vi "setMode.vi"(8 "error in (no error)":errorcluster, 10 "mode":T1, 11 "DmmKeysight in":refnum<class "DmmKeysight.lvclass">) -> (0 "error out":errorcluster, 3 "DmmKeysight out":refnum<class "DmmKeysight.lvclass">)   [LabVIEW 2023, in "DmmKeysight.lvclass"]
doc: "<b>Author:</b> Wolfgang\n<b>Description:</b>Define measurement mode: Voltage, Current, Resistance"
uses:
  DmmKeysight.lvclass
  Data/DmmModes.ctl
  Driver/TypeDef/mode.ctl
  DmmKeysight.lvclass/DmmKeysight.ctl
  Multimeter.lvclass
  Driver/Keysight-34450A.lvlib
  sweDmm.lvlib
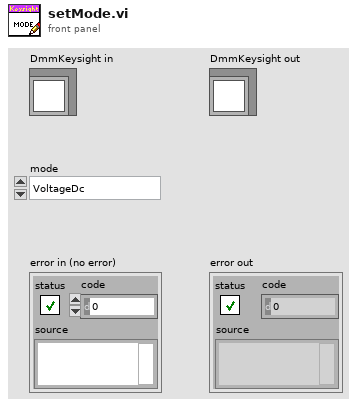
[diagram p1: front panel]
types:
  T1 = typedef "sweDmm.lvlib/DmmModes.ctl" = enum16{"VoltageDc", "VoltageAc", "CurrentDc", "CurrentAc", "Resistance2W"}
  T2 = typedef "Keysight-34450A.lvlib/mode.ctl" = enum16{"DC_Voltage", "AC_Voltage", "DC_Current", "AC_Current", "Resistance"}
  T3 = typedef "Keysight-34450A.lvlib/configuration.ctl" = cluster{"mode":T2, "Range":dbl, "Resolution":dbl}
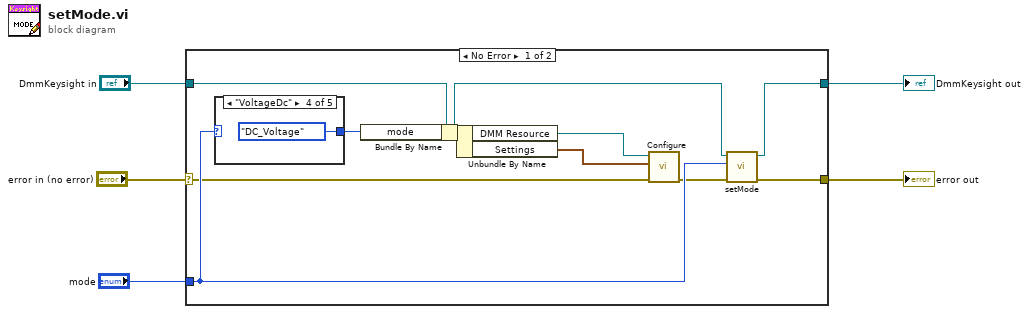
[diagram p0: block diagram]
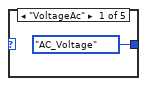
[diagram p2: hidden frame]
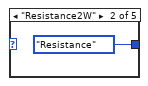
[diagram p3: hidden frame]
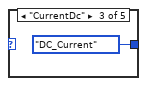
[diagram p4: hidden frame]
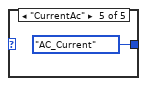
[diagram p5: hidden frame]
diagram:
  n1 = case shown="No Error" "error in (no error)" {
    selector: "error in (no error)" -> [w6 w22]
    tunnel: [w15 w22] -> w5
    tunnel: [w14 w21] -> w4
    tunnel: "DmmKeysight in" -> [w13 w21]
    tunnel: "mode" -> [w12 _]
    frame No Error {
      n2 = case shown="\"VoltageDc\"" w12 {
        tunnel: [mode."AC_Voltage" ("Type") mode."Resistance" ("Type") mode."DC_Current" ("Type") mode."DC_Voltage" ("Type") mode."AC_Current" ("Type")] -> w11
        frame "VoltageAc" {
        }
        frame "Resistance2W" {
        }
        frame "CurrentDc" {
        }
        frame "VoltageDc" {
        }
        frame "CurrentAc" {
        }
      }
      n3 = Bundle By Name(cluster=w13, "mode"=w11) -> (w10:refnum<class "DmmKeysight.lvclass">)
      n4 = Unbundle By Name(w10) -> ("DMM Resource"=w9:refnum<visa-resource-name>, "Settings"=w7:T3)
      n5 = call "Configure.vi"("error in (no error)"=w6, "Configuration"=w7, "VISA resource name"=w9) -> ("error out"=w8:errorcluster)  [unwired: 7 in, 1 out]
      n6 = call-parent "setMode.vi"("error in (no error)"=w8, "Mode"=w12, "Multimeter in"=w10) -> ("error out"=w15:errorcluster, "Multimeter out"=w14:refnum<class "DmmKeysight.lvclass">)  [unwired: 7 in]
    }
    frame Error {
    }
  }
  "error out" <- w5
  "DmmKeysight out" <- w4
